vi "Set Alpha Mask.vi"(6 "Mask?":bool, 8 "error in (no error)":errorcluster, 11 "Car Wash Console in":refnum<class "Car Wash Console.lvclass">) -> (0 "error out":errorcluster, 3 "Car Wash Console out":refnum<class "Car Wash Console.lvclass">)   [LabVIEW 2016, in "CLD Exam - Car Wash.lvlib" / "Car Wash Console.lvclass"]
uses:
  Car Wash Console.lvclass
  Car Wash Console.lvclass/Car Wash Console.ctl
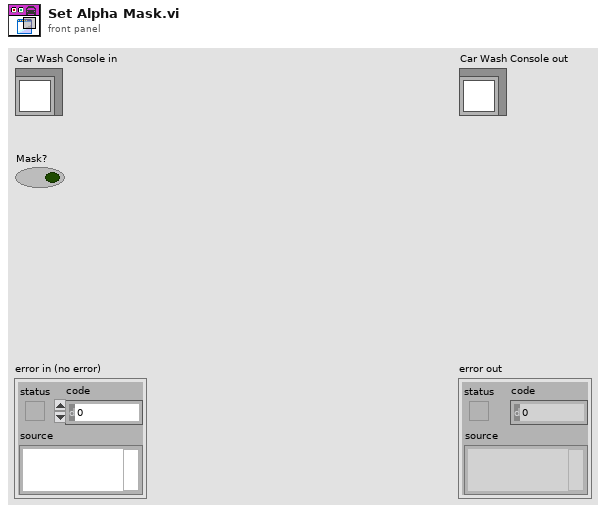
[diagram p1: front panel]
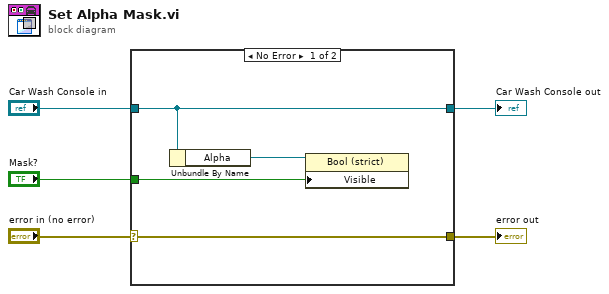
[diagram p0: block diagram]
diagram:
  n1 = case shown="No Error" "error in (no error)" {
    selector: "error in (no error)" -> [w9 w11]
    tunnel: [w9 w11] -> w4
    tunnel: [w8 w10] -> w2
    tunnel: "Car Wash Console in" -> [w8 w10]
    tunnel: "Mask?" -> [w6 _]
    frame No Error {
      n2 = Unbundle By Name(w8) -> ("Alpha"=w7:refnum<vi>)
      n3 = property class="Bool (strict)"(reference=w7, "Visible"=w6) -> ()  [unwired: 1 in, 2 out]
    }
    frame Error {
    }
  }
  "error out" <- w4
  "Car Wash Console out" <- w2
